vi "get top level section in TOML data.vi"(7 "Section name":string caption="Section name (Section data name if empty)", 8 "error in (no error)":errorcluster, 9 "Error if missing element":bool=TRUE caption="Error if missing element (T)", 10 "Section datatype":variant, 11 "Value in":T1) -> (0 "error out":errorcluster, 2 "Missing elements":string[](array[string]), 3 "LV Value":variant)   [LabVIEW 2020, in "TOML.lvlib"]
doc: "Edit a top level element (section) in the TOML data\nMatch the elemnt by \"Section name\""
uses:
  TOML.lvlib
  TOML Value.ctl
  TOML Key-Value Pair.ctl
  <vilib>/ErrorRing/Error Ring.xnode
  <vilib>/Utility/Data Type/NI_Data Type.lvlib
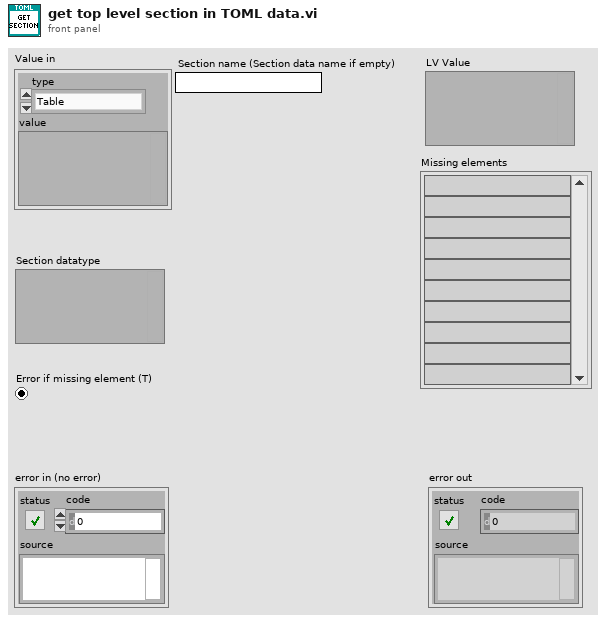
[diagram p1: front panel]
types:
  T1 = typedef "TOML.lvlib/TOML Value.ctl" = cluster{"type":enum16{"Table", "Array", "String", "Integer", "Float", "Boolean", "Offset Date-Time", "Local Date-Time", "Local Date", "Local Time", "Path"}, "value":variant}
  T2 = typedef "TOML.lvlib/TOML Key-Value Pair.ctl" = cluster{"Key":string, "Value":T1}
  T3 = typedef "NI_Data Type.lvlib/Data Type.ctl" = enum8{"Invalid Type", "Void", "I8", "I16", "I32", "I64", "U8", "U16", "U32", "U64", "Single Float", "Double Float", "Extended Float", "Single Complex", "Double Complex", "Extended Complex", "Enum U8", "Enum U16", "Enum U32", "Enum U64", "Single Float With Unit", "Double Float With Unit", "Extended Float With Unit", "Single Complex with Unit", "Double Complex with Unit", "Extended Complex with Unit", "Boolean", "String", "Path", "Picture", "Tag", "Array", "Cluster", "Variant", "LV Variant", "Waveform", "Timestamp", "Digital Waveform", "Digital Data", "ExpressData", "Refnum", "External Data", "VI", "Poly VI", "LabVIEW Class Instance", "Fixed Point", "Set Collection", "Map Collection"}
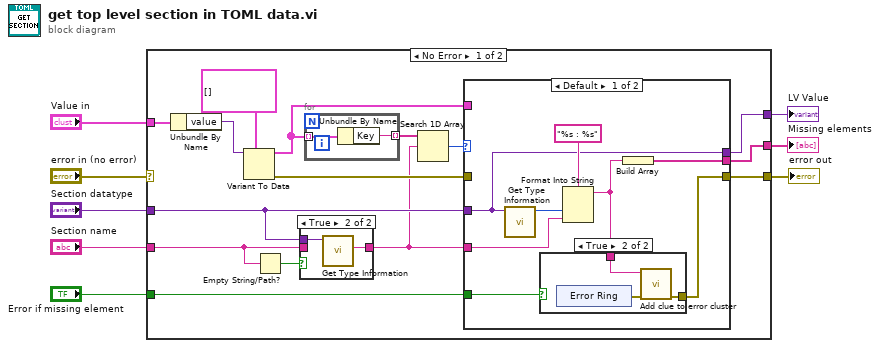
[diagram p0: block diagram]
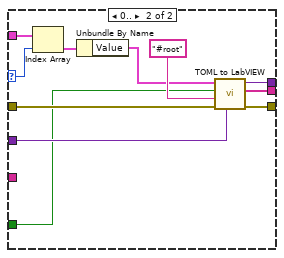
[diagram p4: hidden frame]
diagram:
  n1 = case shown="No Error" "error in (no error)" {
    selector: "error in (no error)" -> [_ w52]
    tunnel: "Value in" -> [w23 _]
    tunnel: "Section datatype" -> [w12 _]
    tunnel: "Section name" -> [w13 _]
    tunnel: [w16 w52] -> w4
    tunnel: [w15 _] -> w3
    tunnel: [w11 _] -> w2
    tunnel: "Error if missing element" -> [w10 _]
    frame No Error {
      n2 = Unbundle By Name(w23) -> ("value"=w22:variant)
      n3 = Variant To Data(type=T2[] [], Variant=w22) -> (data=w19:T2[], error out=w17:errorcluster)  [unwired: 1 in]
      n4 = Empty String/Path?(string/path=w13) -> (empty?=w14:bool)
      n5 = case shown="True" w14 {
        tunnel: w13 -> [w24 _]
        tunnel: [w24 w26] -> w9
        tunnel: w12 -> [_ w25]
        frame False {
        }
        frame True {
          n6 = call <vilib>:"Get Type Information.vi"("variant"=w25) -> ("name"=w26:string)  [unwired: 6 in, 4 out]
        }
      }
      n7 = for {
        tunnel: w19 -> [w51] mode=indexing
        tunnel: [w50] -> w20 mode=indexing
        n8 = Unbundle By Name(w51) -> ("Key"=w50:string)
      }
      n9 = Search 1D Array(1D array=w20, element=w9) -> (index of element=w18:i32)  [unwired: 1 in]
      n10 = case shown="Default" w18 {
        selector: w18 -> [_ w48]
        tunnel: w19 -> [_ w49]
        tunnel: w12 -> [w30 w43]
        tunnel: w17 -> [_ w44]
        tunnel: [w28 w41] -> w16
        tunnel: [w30 w42] -> w15
        tunnel: [w34 w40] -> w11
        tunnel: w10 -> [w27 w39]
        tunnel: w9 -> [w31 _]
        frame Default {
          n11 = call <vilib>:"Get Type Information.vi"("variant"=w30) -> ("type"=w32:T3)  [unwired: 6 in, 4 out]
          n12 = Format Into String(format string="%s : %s", w32, w31) -> (resulting string=w29:string)  [unwired: 2 in, 1 out]
          n13 = case shown="True" w27 {
            tunnel: w29 -> [_ w36]
            tunnel: [_ w35] -> w28
            frame False {
            }
            frame True {
              n14 = xnode "Error Ring"() -> ("error out"=w37:errorcluster)
              n15 = call "Add clue to error cluster.vi"("error in (no error)"=w37, "String"=w36) -> ("error out"=w35:errorcluster)  [unwired: 9 in]
            }
          }
          n16 = Build Array(w29) -> (w34:string[])
        }
        frame 0.. {
          n17 = Index Array(array=w49, index=w48) -> (element=w46:T2)
          n18 = Unbundle By Name(w46) -> ("Value"=w45:T1)
          n19 = call "TOML to LabVIEW.vi"("Default Value"=w43, "error in (no error)"=w44, "Parent"="#root", "Error if missing element"=w39, "TOML Value"=w45) -> ("error out"=w41:errorcluster, "Missing elements"=w40:string[], "LV Value"=w42:variant)  [unwired: 4 in]
        }
      }
    }
    frame Error {
    }
  }
  "error out" <- w4
  "LV Value" <- w3
  "Missing elements" <- w2
